vi "Get_Markers.vi"(8 "Draw?":bool=TRUE, 9 "offset %":dbl=0.2 format="%#_3g", 10 "pixels up":dbl=20.0, 11 "dimensions":i32[](array[numeric])=[2, 3]) -> (1 "last two points":cluster{dbl, dbl}[](array[cluster]), 3 "Edge Points":cluster{dbl, dbl}[][](array[cluster])=[[{0.0, 0.0}, {0.0, 0.0}, {-14.645040518764251, 6.443817828256269}, {-18.306300648455313, 8.054772285320336}, {-32.95134116721957, 14.498590113576606}, {-36.612601296910626, 16.109544570640672}, {0.0, 0.0}, {0.0, 0.0}], [{0.0, 0.0}, {0.0, 0.0}, {14.535847242857194, 6.6864897317143095}, {18.16980905357149, 8.358112164642886}, {32.705656296428685, 15.044601896357197}, {36.33961810714298, 16.716224329285772}, {50.875465350000184, 23.402714061000083}, {54.50942716071448, 25.074336493928662}]])   [LabVIEW 2022 SP3]
panel:
  out "picture out":picture
  # "left line"
  # "right line"
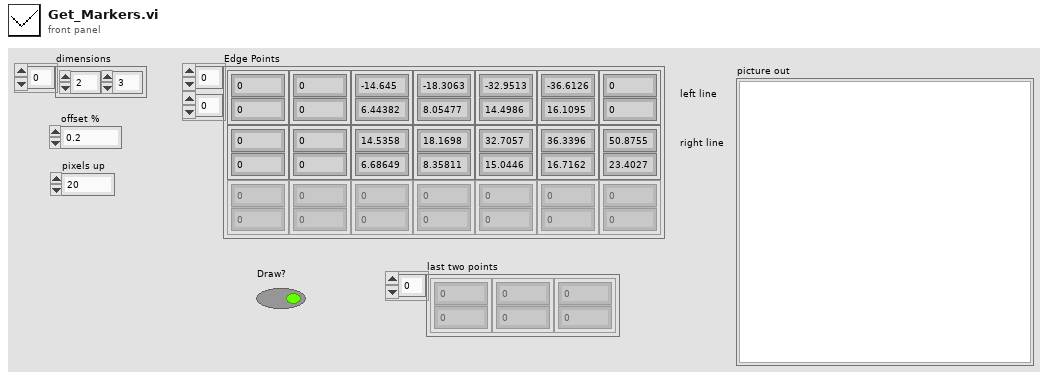
[diagram p1: front panel]
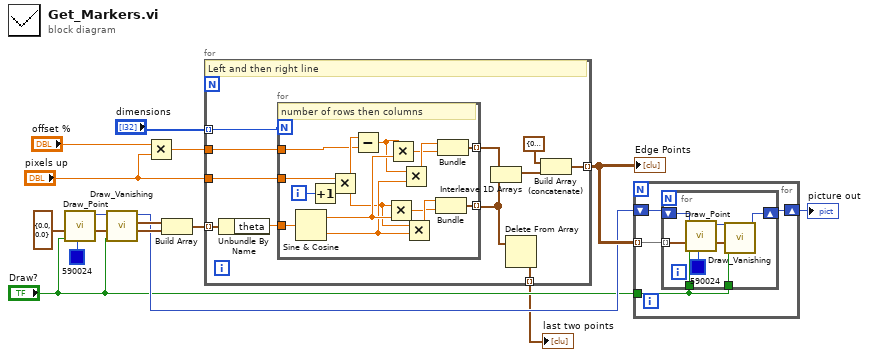
[diagram p0: block diagram]
diagram:
  w4 = cluster{"x":dbl, "y":dbl} {"x"=0.0, "y"=0.0} ("point")
  n1 = call "Draw_Point.vi"("color"=u32 590024, "Draw?"="Draw?", "point"=w4) -> ("new picture"=w3:picture)  [unwired: 8 in]
  n2 = call "Draw_Vanishing.vi"("Draw?"="Draw?", "point"=w4, "picture in"=w3) -> ("right_line"=w13:cluster{"slope":dbl, "b":dbl, "theta":dbl}, "left_line"=w12:cluster{"slope":dbl, "b":dbl, "theta":dbl}, "picture out"=w7:picture)  [unwired: 6 in]
  n3 = Multiply(x="offset %", y="pixels up") -> (x*y=w9:dbl)
  n4 = Build Array(w12, w13) -> (w14:cluster{"slope":dbl, "b":dbl, "theta":dbl}[])
  n5 = for {
    tunnel: "pixels up" -> [w26]
    tunnel: [w18] -> w8 mode=indexing
    tunnel: w14 -> [w24] mode=indexing
    tunnel: "dimensions" -> [w22] mode=indexing
    tunnel: w9 -> [w23]
    tunnel: [w16] -> w1 mode=indexing
    # "Left and then right line"
    n6 = Unbundle By Name(w24) -> ("theta"=w25:dbl)
    n7 = for {
      N: w22 -> [_]
      tunnel: w26 -> [w37]
      tunnel: w25 -> [w41]
      tunnel: [w38] -> w17 mode=indexing
      tunnel: w23 -> [w27]
      tunnel: [w31] -> w20 mode=indexing
      i -> [w36]
      # "number of rows then columns"
      n8 = Sine & Cosine(0:w41) -> (1:w35:dbl, 2:w34:dbl)
      n9 = Increment(x=w36) -> (x+1=w30:i32)
      n10 = Multiply(x=w37, y=w30) -> (x*y=w28:dbl)
      n11 = Subtract(x=w28, y=w27) -> (x-y=w29:dbl)
      n12 = Multiply(x=w28, y=w35) -> (x*y=w39:dbl)
      n13 = Multiply(x=w29, y=w35) -> (x*y=w32:dbl)
      n14 = Multiply(x=w29, y=w34) -> (x*y=w33:dbl)
      n15 = Multiply(x=w28, y=w34) -> (x*y=w40:dbl)
      n16 = Bundle(w40, w39) -> (w38:cluster{dbl, dbl})  [unwired: 1 in]
      n17 = Bundle(w33, w32) -> (w31:cluster{dbl, dbl})  [unwired: 1 in]
    }
    n18 = Interleave 1D Arrays(w20, w17) -> (w19:cluster{dbl, dbl}[])
    n19 = Delete From Array(array=w17) -> (deleted portion=w16:cluster{dbl, dbl})  [unwired: 2 in, 1 out]
    n20 = Build Array (concatenate)(cluster{"x":dbl, "y":dbl} {"x"=0.0, "y"=0.0} ("point"), w19) -> (w18:cluster{"x":dbl, "y":dbl}[])
  }
  "Edge Points" <- w8
  "last two points" <- w1
  n21 = for {
    tunnel: w8 -> [w45] mode=indexing
    shift-right: [w44] -> w6
    shift-left: w7 -> [w43]
    tunnel: "Draw?" -> [w42]
    n22 = for {
      tunnel: w45 -> [w50] mode=indexing
      shift-right: [w52] -> w44
      shift-left: w43 -> [w49]
      tunnel: w42 -> [w47]
      tunnel: w42 -> [w46]
      n23 = call "Draw_Point.vi"("color"=u32 590024, "Draw?"=w46, "point"=w50, "picture in"=w49) -> ("new picture"=w48:picture)  [unwired: 7 in]
      n24 = call "Draw_Vanishing.vi"("Draw?"=w47, "point"=w50, "picture in"=w48) -> ("picture out"=w52:picture)  [unwired: 6 in, 2 out]
    }
  }
  "picture out" <- w6
